vi "hw8p8_hickey.vi"() -> ()   [LabVIEW 2014]
uses:
  <vilib>/imath/engines/lvmath2/RunTimeEngine/Managers/WorkSpace/UID Generator.vi
  <vilib>/imath/engines/lvmath2/RunTimeEngine/RunTimeType/NIMS_RunTimeType_From StrictType (excl LVString).vi
  <instcachedir>/0/NIMS_RunTimeType_From StrictType (excl LVString)_15A5391EEA9C4AACB9955AC755B83D29.lvgen/NIMS_RunTimeType_From StrictType (excl LVString)_15A5391EEA9C4AACB9955AC755B83D29_000.vi
  <vilib>/imath/engines/lvmath2/RunTimeEngine/LocalVariableDefStatement/MC_LocalVariableDefStatement_Display.vi
  <vilib>/imath/engines/lvmath2/RunTimeEngine/Managers/SymbolTable/Clear UID.vi
  <vilib>/imath/engines/lvmath2/RunTimeEngine/NodeEndStatement/NIMS_NodeEndStatement_Output.vi
  <instcachedir>/0/NIMS_NodeEndStatement_Output_53EC0D466D134D7ABD903AC30B43404B.lvgen/NIMS_NodeEndStatement_Output_53EC0D466D134D7ABD903AC30B43404B_001.vi
  <vilib>/imath/engines/lvmath2/RunTimeEngine/ErrorHandling/NIMS_Finalize Error.vi
  <vilib>/imath/engines/lvmath2/RunTimeEngine/Managers/SymbolTable/NIMS_WorkSpace.lvlib
panel:
  out "Waveform Graph":dbl[](graph)
  in  "Alpha":dbl
  in  "Numeric":i32
  # "Alpha=.00092 max 103 m/s at 40s"
  # "Alpha=.0035 max of 52.5 m/s at 20s"
  # "Alpha=.11 max of 9.5 m/s at 3.5s"
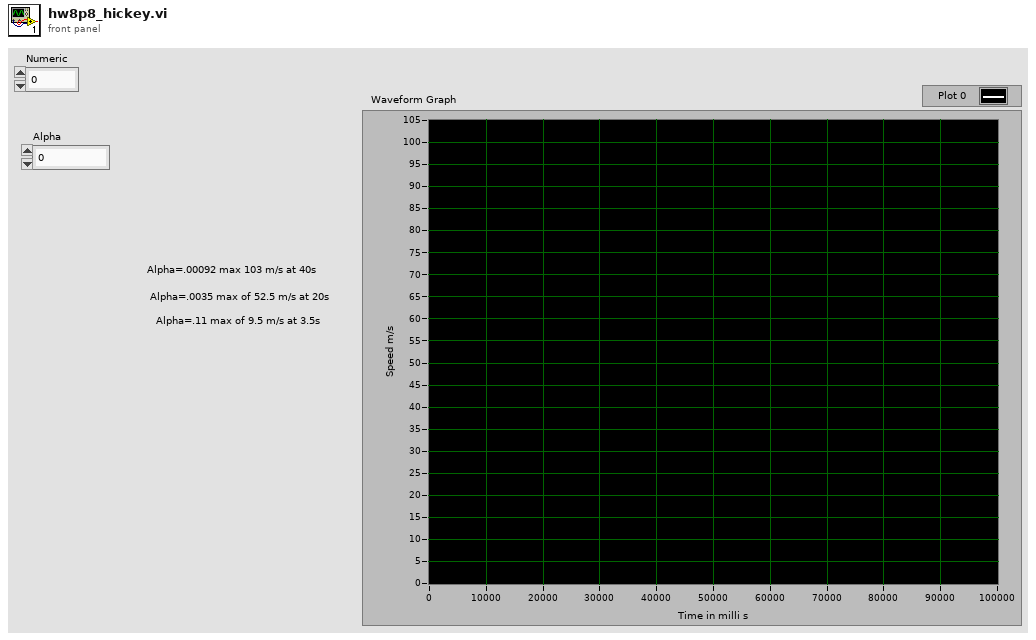
[diagram p1: front panel]
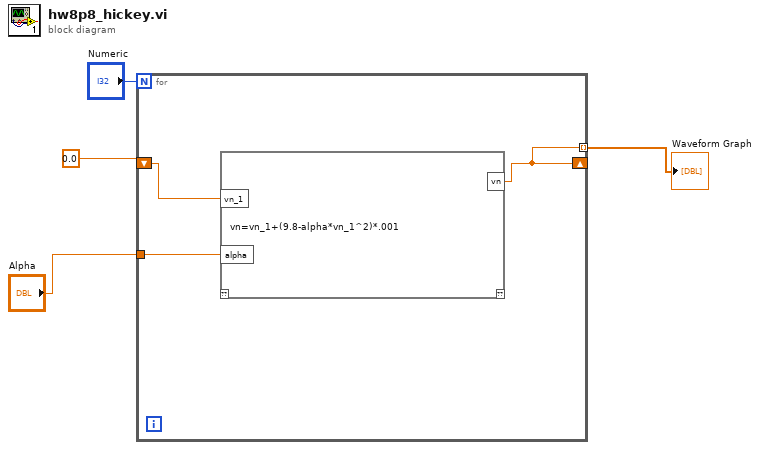
[diagram p0: block diagram]
diagram:
  n1 = for {
    N: "Numeric" -> [_]
    shift-right: [w5] -> _
    shift-left: 0.0 -> [w7]
    tunnel: "Alpha" -> [w6]
    tunnel: [w5] -> w1 mode=indexing
    n2 = mathscript code="vn=vn_1+(9.8-alpha*vn_1^2)*.001"("vn_1"=w7, "alpha"=w6) -> ("vn"=w5:dbl)  [unwired: 1 in, 1 out]
  }
  "Waveform Graph" <- w1
